vi "Stop Form Server.vi"(8 "error in (no error)":errorcluster, 11 "Form Server Wrapper in":refnum<class "Form Server Wrapper.lvclass">) -> (0 "error out":errorcluster)   [LabVIEW 2020, in "Form Server.lvlib" / "Form Server Wrapper.lvclass"]
uses:
  Form Server Wrapper.lvclass
  Form Server Wrapper.lvclass/Form Server Wrapper.ctl
  <vilib>/ActorFramework/Message Enqueuer/Message Enqueuer.lvclass/Message Enqueuer.ctl
  <vilib>/ActorFramework/Message Enqueuer/Enqueue.vi
  <vilib>/ActorFramework/Stop Msg/Stop Msg.lvclass
  C:/Program Files (x86)/National Instruments/LabVIEW 2020/vi.lib/ActorFramework/Message/Message.lvclass
  <vilib>/ActorFramework/Message Priority Queue/Priority Enqueue.vi
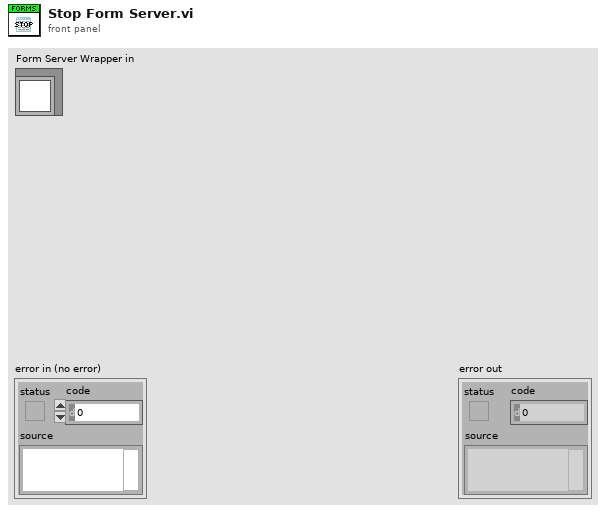
[diagram p1: front panel]
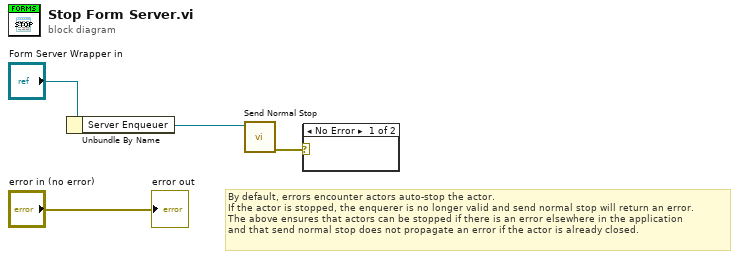
[diagram p0: block diagram]
diagram:
  # "By default, errors encounter actors auto-stop the actor.\nIf the actor is stopped, the enquerer is no longer valid and send normal stop will return an error.\nThe above ensures that actors can be stopped if there is an error elsewhere in the application\nand that send normal stop does not propagate an error if the actor is already closed."
  n1 = Unbundle By Name("Form Server Wrapper in") -> ("Server Enqueuer"=w3:refnum<class "Message Enqueuer.lvclass">)
  n2 = call <vilib>:"Send Normal Stop.vi"("Message Enqueuer"=w3) -> ("error out"=w1:errorcluster)  [unwired: 10 in]
  n3 = case shown="No Error" w1 {
    frame No Error {
    }
    frame Error {
    }
  }
  "error out" <- "error in (no error)"
